vi "Pre Launch Init.vi"(11 "上位机代理者 in":refnum<class "服务器.lvclass"> caption="操作者输入") -> (0 "error out":errorcluster caption="错误输出", 3 "上位机代理者 out":refnum<class "服务器.lvclass"> caption="操作者输出")   [LabVIEW 2015, in "服务器.lvlib" / "服务器.lvclass"]
doc: "(<B>Filename</B>: Actor Framework.lvlib:Actor.lvclass:Pre Launch Init.vi)\n\nDefines behavior that occurs after the Launch Nested Actor method is invoked but before the actor's Actor Core method begins running.\n\nBy default, this method does nothing. A descendant class may override it to define behavior."
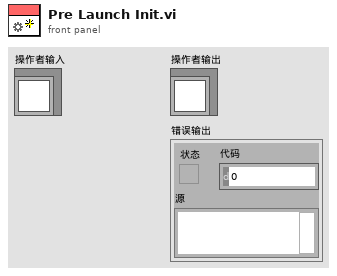
[diagram p1: front panel]
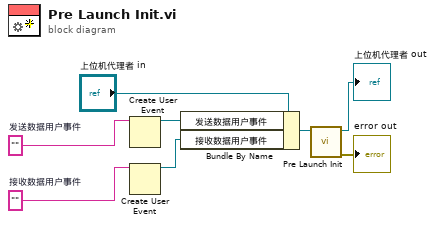
[diagram p0: block diagram]
diagram:
  w5 = ""  # 接收数据用户事件
  w6 = ""  # 发送数据用户事件
  n1 = Create User Event(user event datatype=w6) -> (user event=w3:refnum<user-event>)  [unwired: 1 in, 1 out]
  n2 = Create User Event(user event datatype=w5) -> (user event=w4:refnum<user-event>)  [unwired: 1 in, 1 out]
  n3 = Bundle By Name(cluster="上位机代理者 in", "发送数据用户事件"=w3, "接收数据用户事件"=w4) -> (w1:refnum<class "服务器.lvclass">)
  n4 = call-parent "Pre Launch Init.vi"("前面板控制 in"=w1) -> ("error out"=→"error out":errorcluster, "前面板控制 out"=→"上位机代理者 out":refnum<class "服务器.lvclass">)  [unwired: 9 in]
